vi "Create Groups.vi"(8 "error in (no error)":errorcluster, 9 "framework options":T1={"FIFO Options"={"Infinite Timeouts"=FALSE}, "Thread Options"={"Show FP On Call"=FALSE, "Close FP After Call"=FALSE, "Allow Debugging"=FALSE}, "Plugin Options"={"Default Components"=FALSE}, "Performance Options"={"Measure Period"=FALSE, "Measure Rx/Tx Duration"=FALSE}, "Data Server Options"={"Enable Data Server"=FALSE, "Period"=50}} {"Data Server Options"."Period" format="%d ms"}, 10 "Framework Configuration":refnum<class "Framework Configuration.lvclass">, 11 "Framework in":refnum<class "Framework.lvclass">) -> (0 "error out":errorcluster, 2 "Transfer Groups":refnum<class "Transfer Group.lvclass">[](array[class]), 3 "Framework out":refnum<class "Framework.lvclass">)   [LabVIEW 2021, in "DSF Core.lvlib" / "Framework.lvclass"]
uses:
  Framework.lvclass
  Configuration/Core/Framework/Framework Configuration.lvclass
  Transfer Group/Transfer Group.lvclass
  Framework Options.ctl
  Typedefs/DSF FIFO Options.ctl
  Thread/Thread Options.ctl
  Typedefs/DSF Plugin Options.ctl
  Typedefs/DSF Performance Options.ctl
  Data Server Options.ctl
  Configuration/Core/Plugin/Plugin Configuration.lvclass
  Configuration/Core/Thread/Thread Configuration.lvclass
  Thread/Thread.lvclass
  DSF Core.lvlib
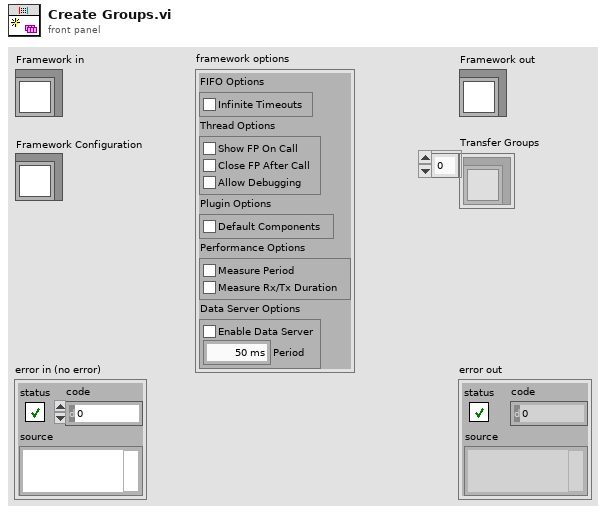
[diagram p1: front panel]
types:
  T1 = typedef "DSF Core.lvlib/Framework.lvclass/Framework Options.ctl" = cluster{"FIFO Options":T2, "Thread Options":T3, "Plugin Options":T4, "Performance Options":T5, "Data Server Options":T6}
  T2 = typedef "DSF Core.lvlib/Framework.lvclass/DSF FIFO Options.ctl" = cluster{"Infinite Timeouts":bool}
  T3 = typedef "DSF Core.lvlib/Thread.lvclass/Thread Options.ctl" = cluster{"Show FP On Call":bool, "Close FP After Call":bool, "Allow Debugging":bool}
  T4 = typedef "DSF Core.lvlib/Framework.lvclass/DSF Plugin Options.ctl" = cluster{"Default Components":bool}
  T5 = typedef "DSF Core.lvlib/DSF Performance Options.ctl" = cluster{"Measure Period":bool, "Measure Rx/Tx Duration":bool}
  T6 = typedef "DSF Core.lvlib/Framework.lvclass/Data Server Options.ctl" = cluster{"Enable Data Server":bool, "Period":u32}
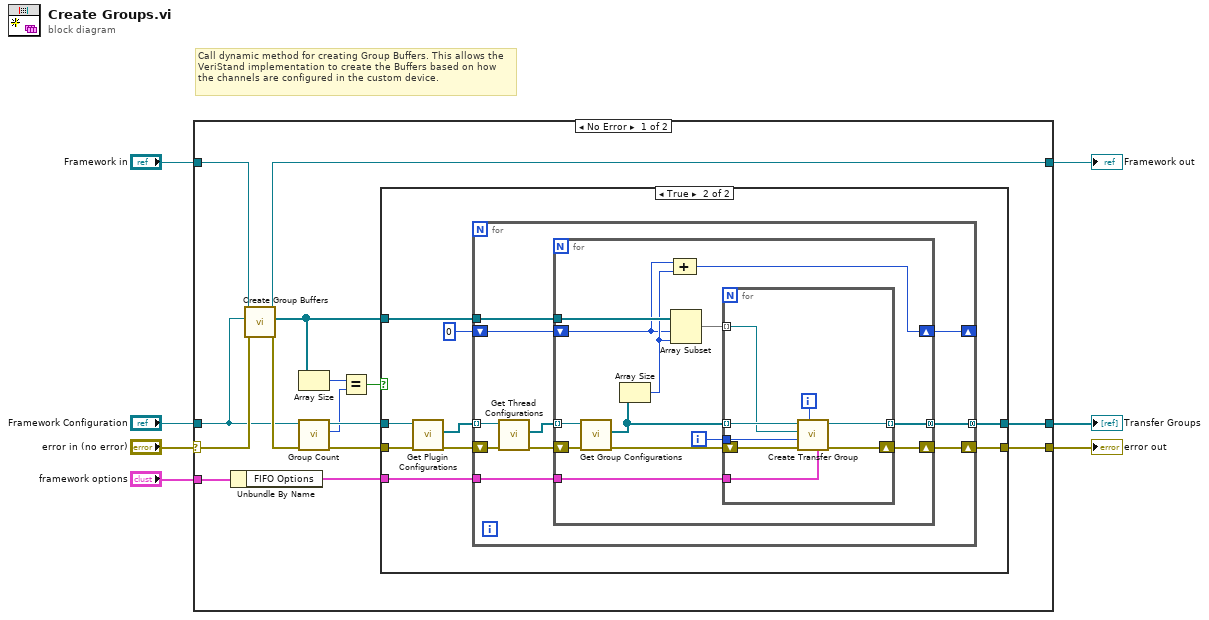
[diagram p0: block diagram]
diagram:
  # "Call dynamic method for creating Group Buffers. This allows the VeriStand implementation to create the Buffers based on how the channels are configured in the custom device."
  n1 = case shown="No Error" "error in (no error)" {
    selector: "error in (no error)" -> [w18 w65]
    tunnel: [w21 w65] -> w6
    tunnel: [w19 w64] -> w4
    tunnel: "Framework in" -> [w20 w64]
    tunnel: "Framework Configuration" -> [w15 _]
    tunnel: [w22 _] -> w2
    tunnel: "framework options" -> [w9 _]
    frame No Error {
      n2 = Unbundle By Name(w9) -> ("FIFO Options"=w8:T2)
      n3 = call-dynamic "Create Group Buffers.vi"("error in (no error)"=w18, "Framework Configuration"=w15, "Framework in"=w20) -> ("error out"=w17:errorcluster, "Group Buffers"=w14:refnum<class "Buffers.lvclass">[], "Framework out"=w19:refnum<class "Framework.lvclass">)  [unwired: 6 in]
      n4 = Array Size(array=w14) -> (size(s)=w13:i32)
      n5 = call-dynamic "Group Count.vi"("error in (no error)"=w17, "Framework Configuration in"=w15) -> ("error out"=w16:errorcluster, "group count"=w11:i32, "Framework Configuration out"=w12:refnum<class "Framework Configuration.lvclass">)  [unwired: 7 in]
      n6 = Equal?(x=w13, y=w11) -> (x = y?=w10:bool)
      n7 = case shown="True" w10 {
        tunnel: [_ w30] -> w22
        tunnel: [w23 w29] -> w21
        tunnel: w14 -> [_ w28]
        tunnel: w16 -> [w23 w26]
        tunnel: w12 -> [_ w25]
        tunnel: w8 -> [_ w24]
        frame False {
          # "#TODO\nError. Buffers count does not match configured Group count."
        }
        frame True {
          n8 = call "Get Plugin Configurations.vi"("error in (no error)"=w26, "Framework Configuration in"=w25) -> ("error out"=w31:errorcluster, "Plugin Configurations"=w32:refnum<class "Plugin Configuration.lvclass">[])  [unwired: 7 in, 1 out]
          n9 = for {
            tunnel: w32 -> [w42] mode=indexing
            shift-right: [w37] -> w29
            shift-left: w31 -> [w40]
            tunnel: [w38] -> w30 mode=concatenating
            tunnel: w28 -> [w36]
            shift-right: [w34] -> _
            shift-left: 0 ("size(s)") -> [w35]
            tunnel: w24 -> [w33]
            n10 = call "Get Thread Configurations.vi"("error in (no error)"=w40, "Plugin Configuration in"=w42) -> ("error out"=w39:errorcluster, "Thread Configurations"=w41:refnum<class "Thread Configuration.lvclass">[])  [unwired: 7 in, 1 out]
            n11 = for {
              tunnel: w41 -> [w55] mode=indexing
              shift-right: [w51] -> w37
              shift-left: w39 -> [w54]
              tunnel: [w52] -> w38 mode=concatenating
              tunnel: w36 -> [w49]
              shift-right: [w45] -> w34
              shift-left: w35 -> [w46]
              tunnel: w33 -> [w44]
              i -> [w43]
              n12 = call "Get Group Configurations.vi"("error in (no error)"=w54, "Thread Configuration in"=w55) -> ("error out"=w53:errorcluster, "Group Configurations"=w50:refnum<class "Group Configuration.lvclass">[])  [unwired: 7 in, 1 out]
              n13 = Array Size(array=w50) -> (size(s)=w47:i32)
              n14 = Array Subset(array=w49, index=w46, length=w47) -> (w48:refnum<class "Buffers.lvclass">[])
              n15 = Compound Arithmetic op=ADD(w46, w47) -> (w45:i32)
              n16 = for {
                tunnel: w50 -> [w59] mode=indexing
                shift-right: [w62] -> w51
                shift-left: w53 -> [w60]
                tunnel: [w63] -> w52 mode=indexing
                tunnel: w48 -> [w58] mode=indexing
                tunnel: w44 -> [w57]
                tunnel: w43 -> [w56]
                i -> [w61]
                n17 = call "Create Transfer Group.vi"("FIFO options"=w57, "id (0)"=w61, "error in"=w60, "thread index"=w56, "buffers"=w58, "group configuration"=w59) -> ("error out"=w62:errorcluster, "transfer group out"=w63:refnum<class "Transfer Group.lvclass">)  [unwired: 4 in]
              }
            }
          }
        }
      }
    }
    frame Error {
    }
  }
  "error out" <- w6
  "Framework out" <- w4
  "Transfer Groups" <- w2
